vi "add_uint8.vi"   [LabVIEW 2010]
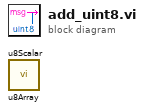
[diagram p0: block diagram]
diagram:
  n1 = call <userlib>:"u8Array.vi"() -> ()  [unwired: 5 in, 1 out]
  n2 = call <userlib>:"u8Scalar.vi"() -> ()  [unwired: 5 in, 1 out]
